vi "Main.vi"(5 "Deliminated Char":string=".", 6 "Folder names":string[](array[string])=["StaARx#[PLC]StaATesterRxSignals", "StaATx#[PLC]StaATesterTxSignals"], 7 "PLC FGVname":string="OPC Ref", 8 "error in":errorcluster, 9 "Sequence Context In":refnum<k7>, 10 "Event Sources":T1, 11 "PreUUT In":refnum<class "PreUUT.lvclass">) -> (0 "error out":errorcluster, 2 "Station":string="asdfasdf", 3 "OPC UA Out":refnum<class "PreUUT.lvclass">)   [LabVIEW 2021, in "OPC UA.lvlib" / "PreUUT.lvclass"]
uses:
  PreUUT.lvclass
  Controls/Rx PreUUT.ctl
  Controls/Tx PreUUT.ctl
  PreUUT.lvclass/PreUUT.ctl
  <vilib>/addons/TestStand/_TSUtility.llb/TestStand - Get Property Value (Number {Signed 32-bit Integer}).vi
  OPC UA/OPC UA.lvclass
panel:
  in  "Terminate":bool
  out "Connect?":bool
  in  "Tx PreUUT":T2={"Online"=TRUE, "Ready"=TRUE, "Fault"=FALSE, "Timeout"=FALSE, "Results"=0, "StepNo"=0, "TestRunning"=FALSE, "ResultsReady"=FALSE, "Heartbeat"=FALSE}
  out "Rx PreUUT":T3
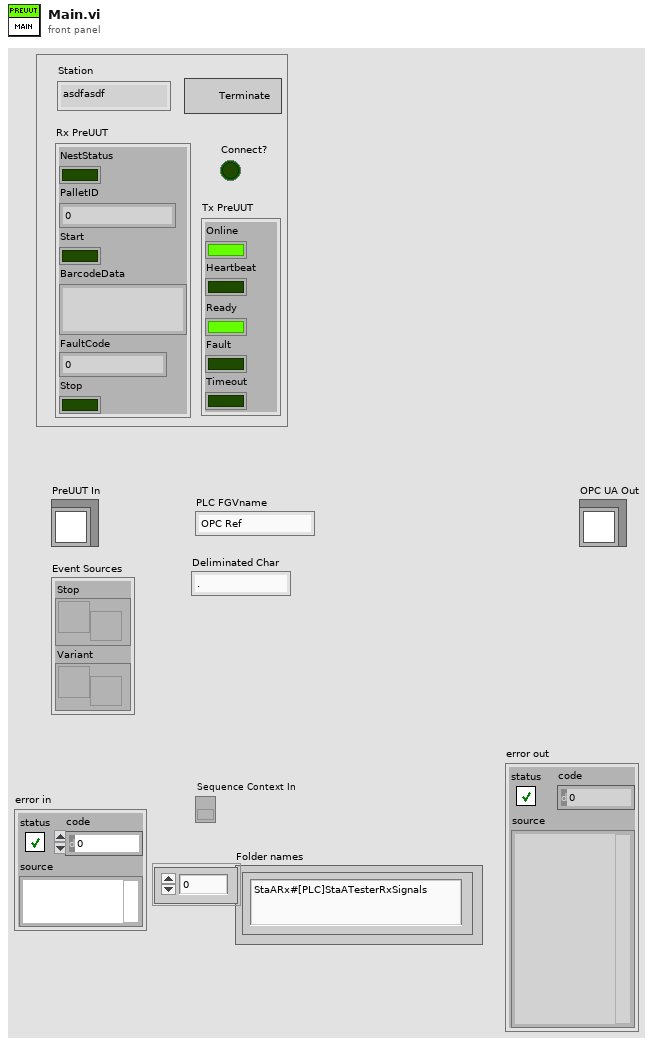
[diagram p1: front panel]
types:
  T1 = cluster{"Stop":refnum<user-event>, "Variant":refnum<user-event>}
  T2 = typedef "OPC UA.lvlib/PreUUT.lvclass/Tx PreUUT.ctl" = cluster{"Online":bool, "Ready":bool, "Fault":bool, "Timeout":bool, "Results":u32, "StepNo":u32, "TestRunning":bool, "ResultsReady":bool, "Heartbeat":bool}
  T3 = typedef "OPC UA.lvlib/PreUUT.lvclass/Rx PreUUT.ctl" = cluster{"NestStatus":bool, "PalletID":u32, "Start":bool, "BarcodeData":string, "FaultCode":u32, "Stop":bool}
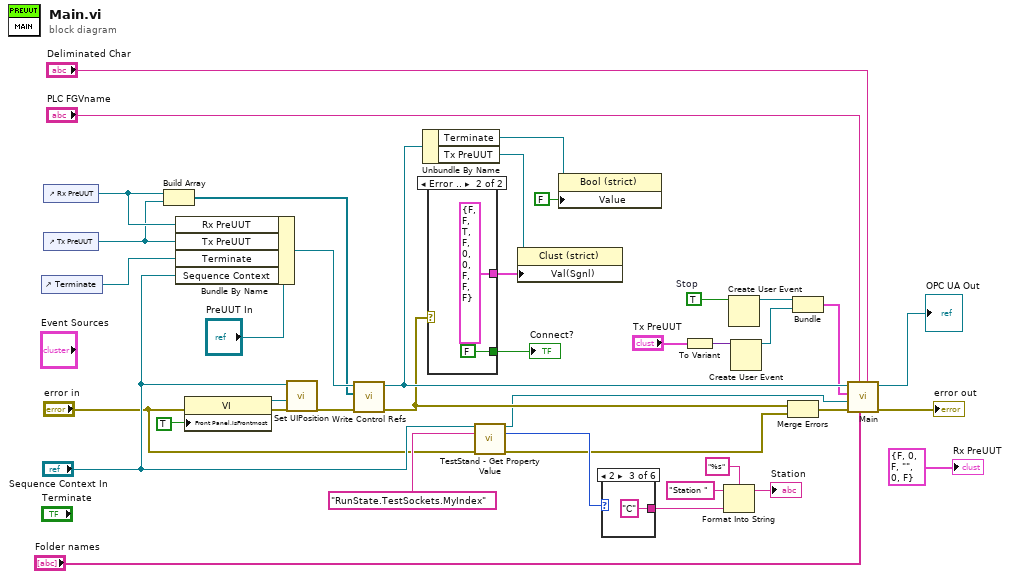
[diagram p0: block diagram]
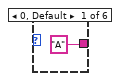
[diagram p2: hidden frame]
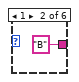
[diagram p3: hidden frame]
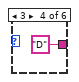
[diagram p4: hidden frame]
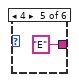
[diagram p5: hidden frame]
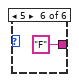
[diagram p6: hidden frame]
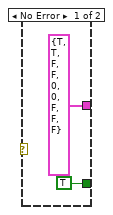
[diagram p7: hidden frame]
diagram:
  w28 = TRUE  # Stop
  n1 = control-ref of="Terminate"() -> (w3:refnum<vi>)
  n2 = control-ref of="Rx PreUUT"() -> (w35:refnum<vi>)
  n3 = control-ref of="Tx PreUUT"() -> (w34:refnum<vi>)
  n4 = Build Array(w35, w34) -> (w33:refnum<vi>[])
  n5 = Bundle By Name(cluster="PreUUT In", "Rx PreUUT"=w35, "Tx PreUUT"=w34, "Terminate"=w3, "Sequence Context"="Sequence Context In") -> (w36:refnum<class "PreUUT.lvclass">)
  n6 = property class="VI"(error in="error in", "Front Panel.IsFrontmost"=TRUE ("Front Panel Window:Is Frontmost")) -> (reference out=w20:refnum<vi>, error out=w21:errorcluster)  [unwired: 1 in]
  n7 = call "Set UIPosition.vi"("error in"=w21, "VI Ref"=w20, "Sequence Context In"="Sequence Context In") -> ("error out"=w22:errorcluster)  [unwired: 8 in]
  n8 = call-dynamic "Write Control Refs.vi"("error in (no error)"=w22, "Ctl Refs"=w33, "OPC UA in"=w36) -> ("error out"=w5:errorcluster, "OPC UA out"=w25:refnum<class "PreUUT.lvclass">)  [unwired: 7 in]
  n9 = Unbundle By Name(w25) -> ("Terminate"=w2:refnum<vi>, "Tx PreUUT"=w38:refnum<vi>)
  n10 = case shown="Error .." w5 {
    tunnel: [T2 {"Online"=TRUE, "Ready"=TRUE, "Fault"=FALSE, "Timeout"=FALSE, "Results"=0, "StepNo"=0, "TestRunning"=FALSE, "ResultsReady"=FALSE, "Heartbeat"=FALSE} ("Tx PreUUT") T2 {"Online"=FALSE, "Ready"=FALSE, "Fault"=TRUE, "Timeout"=FALSE, "Results"=0, "StepNo"=0, "TestRunning"=FALSE, "ResultsReady"=FALSE, "Heartbeat"=FALSE} ("Tx PreUUT")] -> w39
    tunnel: [TRUE ("Connect?") FALSE ("Connect?")] -> w23
    frame No Error {
    }
    frame Error {
    }
  }
  "Connect?" <- w23
  n11 = call-poly <vilib>:"TestStand - Get Property Value.vi"("Sequence Context In"="Sequence Context In", "Lookup String"="RunState.TestSockets.MyIndex", "error in (no error)"="error in") -> ("Sequence Context Out"=w4:refnum<k7>, "Value"=w14:i32, "error out"=w9:errorcluster)  [unwired: 10 in]
  n12 = property class="Clust (strict)"(reference=w38, "Val(Sgnl)"=w39) -> ()  [unwired: 1 in, 2 out]
  n13 = property class="Bool (strict)"(reference=w2, "Value"=FALSE) -> ()  [unwired: 1 in, 2 out]
  n14 = case shown="2" w14 {
    tunnel: ["A" ("format string") "B" ("format string") "C" ("format string") "D" ("format string") "E" ("format string") "F" ("format string")] -> w15
    frame 0, Default {
    }
    frame 1 {
    }
    frame 2 {
    }
    frame 3 {
    }
    frame 4 {
    }
    frame 5 {
    }
  }
  n15 = To Variant(anything="Tx PreUUT") -> (Variant=w30:variant)
  n16 = Format Into String(format string="%s", initial string="Station ", w15) -> (resulting string=→"Station":string)  [unwired: 1 in, 1 out]
  n17 = Create User Event(user event datatype=w28) -> (user event=w27:refnum<user-event>)  [unwired: 1 in, 1 out]
  n18 = Create User Event(user event datatype=w30) -> (user event=w29:refnum<user-event>)  [unwired: 1 in, 1 out]
  n19 = Merge Errors(w5, w9) -> (w6:errorcluster)
  n20 = Bundle("Stop"=w27, "Variant"=w29) -> (w18:T1)  [unwired: 1 in]
  n21 = call-parent "Main.vi"("Deliminated Char"="Deliminated Char", "Folder names"="Folder names", "FGVname"="PLC FGVname", "error in"=w6, "Sequence Context In"=w4, "Event Sources"=w18, "OPC UA In"=w25) -> ("error out"=→"error out":errorcluster, "OPC UA Out"=→"OPC UA Out":refnum<class "PreUUT.lvclass">)  [unwired: 2 in, 1 out]
  "Rx PreUUT" <- T3 {"NestStatus"=FALSE, "PalletID"=0, "Start"=FALSE, "BarcodeData"="", "FaultCode"=0, "Stop"=FALSE} ("Rx PreUUT")
